vi "Table_Sort.vi"(7 "Sort Type":enum16{"numerical", "hex", "string"}(ring), 9 "Sort by":u16(ring) items=["Packet_Number", "Timestamp", "Source", "Destination", "Protocol", "Length", "Data"], 11 "Unsorted Data":string[][](array[string])=array1500x8[12000 elements]) -> (3 "Sorted data":string[][](array[string]))   [LabVIEW 2025, in "Table_Filtering.lvlib"]
uses:
  Table_Filtering.lvlib
  dd903b07-9a56-4d29-89d8-b4a603456dcb.vi
  <vilib>/Array/Sort 2D Array - Pop Stack.vi
  <vilib>/Array/Sort 2D Array - Push Stack.vi
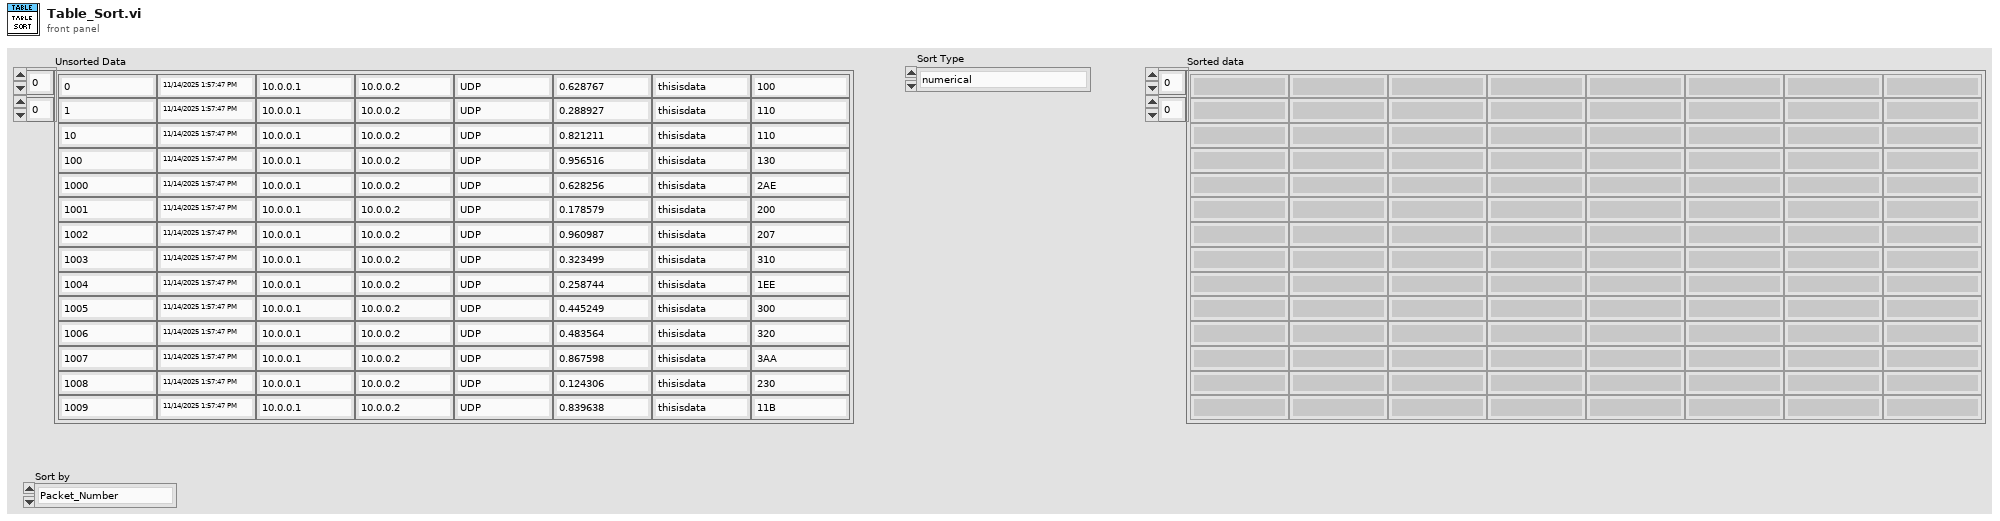
[diagram p1: front panel]
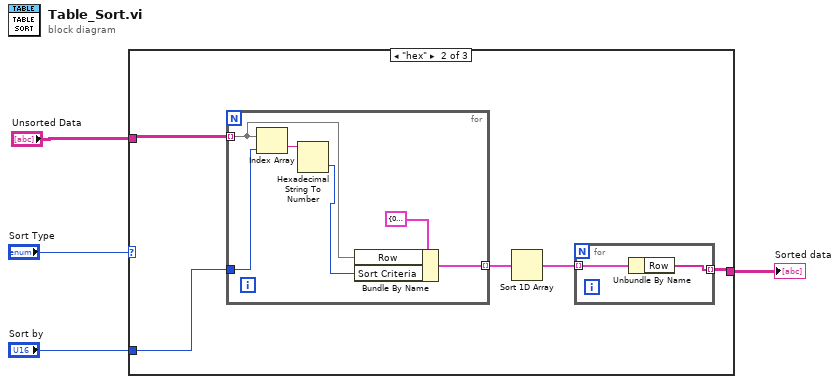
[diagram p0: block diagram]
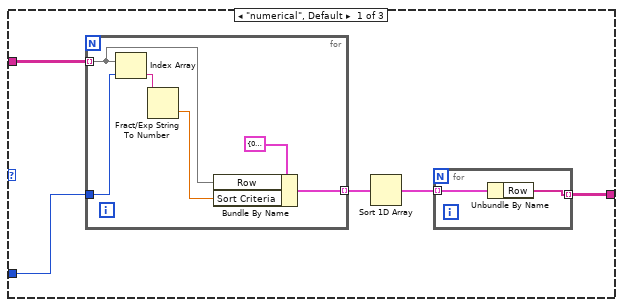
[diagram p2: hidden frame]
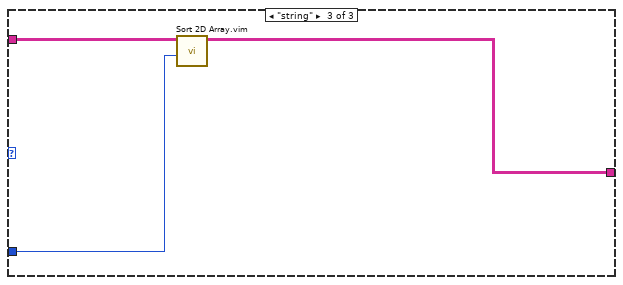
[diagram p3: hidden frame]
diagram:
  n1 = case shown="\"hex\"" "Sort Type" {
    tunnel: "Unsorted Data" -> [w9 w18 w33]
    tunnel: "Sort by" -> [w8 w19 w31]
    tunnel: [w5 w20 w32] -> w2
    frame "numerical", Default {
      n2 = for {
        tunnel: w9 -> [w14] mode=indexing
        tunnel: w8 -> [w15]
        tunnel: [w12] -> w7 mode=indexing
        n3 = Index Array(array=w14, index=w15) -> (element=w17:string)
        n4 = Fract/Exp String To Number(string=w17) -> (number=w13:dbl)  [unwired: 3 in, 1 out]
        n5 = Bundle By Name(cluster=cluster{"Sort Criteria":dbl, "Row":string[]} {"Sort Criteria"=0.0, "Row"=[]}, "Row"=w14, "Sort Criteria"=w13) -> (w12:cluster{"Sort Criteria":dbl, "Row":string[]})
      }
      n6 = Sort 1D Array(array=w7) -> (sorted array=w6:cluster{"Sort Criteria":dbl, "Row":string[]}[])
      n7 = for {
        tunnel: w6 -> [w11] mode=indexing
        tunnel: [w10] -> w5 mode=indexing
        n8 = Unbundle By Name(w11) -> ("Row"=w10:string[])
      }
    }
    frame "hex" {
      n9 = for {
        tunnel: w18 -> [w28] mode=indexing
        tunnel: w19 -> [w29]
        tunnel: [w27] -> w22 mode=indexing
        n10 = Index Array(array=w28, index=w29) -> (element=w26:string)
        n11 = Hexadecimal String To Number(string=w26) -> (number=w25:u32)  [unwired: 2 in, 1 out]
        n12 = Bundle By Name(cluster=cluster{"Sort Criteria":dbl, "Row":string[]} {"Sort Criteria"=0.0, "Row"=[]}, "Row"=w28, "Sort Criteria"=w25) -> (w27:cluster{"Sort Criteria":dbl, "Row":string[]})
      }
      n13 = Sort 1D Array(array=w22) -> (sorted array=w21:cluster{"Sort Criteria":dbl, "Row":string[]}[])
      n14 = for {
        tunnel: w21 -> [w24] mode=indexing
        tunnel: [w23] -> w20 mode=indexing
        n15 = Unbundle By Name(w24) -> ("Row"=w23:string[])
      }
    }
    frame "string" {
      n16 = call "Sort 2D Array.vim"("index"=w31, "2D array"=w33) -> ("sorted 2D array"=w32:string[][])  [unwired: 8 in, 1 out]
    }
  }
  "Sorted data" <- w2
